vi "WPI_MotorControlScaleFromPWM.vi"(10 "Raw PWM Value":u8, 11 "DeadBand Info":T1={"Name"="", "maxPositivePwm"=0, "minPositivePwm"=0, "centerPwm"=0, "maxNegativePwm"=0, "minNegativePwm"=0, "angularRange"=170}) -> (2 "Output (1,-1)":dbl)   [LabVIEW 2017]
doc: "This software is licensed. Open the labview\\readme\\WPI Robotics Library Open Source License.txt file for more information."
uses:
  <vilib>/Rock Robotics/WPI/PWM/WPI_PWMDeadband.ctl
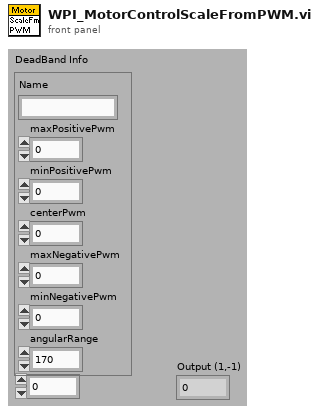
[diagram p1: front panel]
types:
  T1 = typedef "WPI_PWMDeadband.ctl" = cluster{"Name":string, "maxPositivePwm":i32, "minPositivePwm":i32, "centerPwm":i32, "maxNegativePwm":i32, "minNegativePwm":i32, "angularRange":u16}
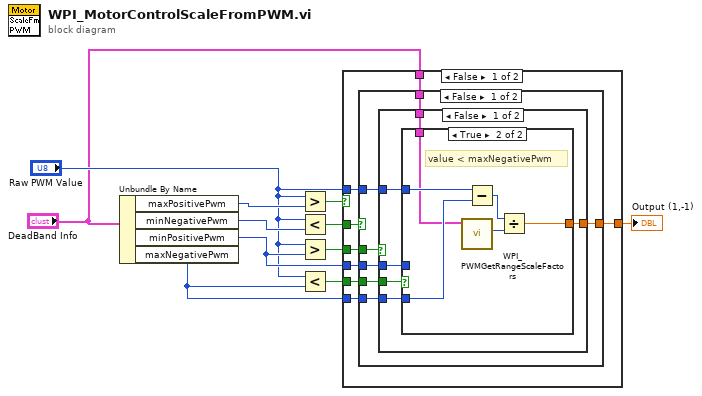
[diagram p0: block diagram]
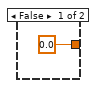
[diagram p2: hidden frame]
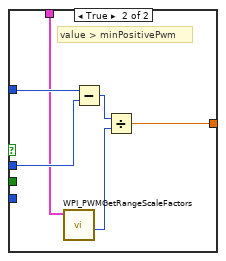
[diagram p3: hidden frame]
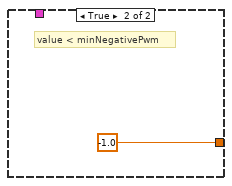
[diagram p4: hidden frame]
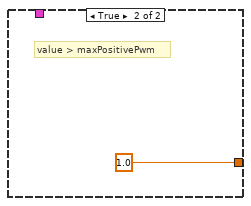
[diagram p5: hidden frame]
diagram:
  n1 = Unbundle By Name("DeadBand Info") -> ("maxPositivePwm"=w11:i32, "minNegativePwm"=w10:i32, "minPositivePwm"=w9:i32, "maxNegativePwm"=w8:i32)
  n2 = Greater?(x="Raw PWM Value", y=w11) -> (0:w4:bool)
  n3 = Less?(x="Raw PWM Value", y=w10) -> (x < y?=w5:bool)
  n4 = Greater?(x="Raw PWM Value", y=w9) -> (0:w6:bool)
  n5 = Less?(x="Raw PWM Value", y=w8) -> (x < y?=w7:bool)
  n6 = case shown="False" w4 {
    tunnel: "Raw PWM Value" -> [w19 _]
    tunnel: w9 -> [w18 _]
    tunnel: "DeadBand Info" -> [w17 _]
    tunnel: w8 -> [w16 _]
    tunnel: [w15 1.0] -> w1
    tunnel: w7 -> [w14 _]
    tunnel: w6 -> [w13 _]
    tunnel: w5 -> [w12 _]
    frame False {
      n7 = case shown="False" w12 {
        tunnel: w19 -> [w26 _]
        tunnel: w18 -> [w25 _]
        tunnel: w17 -> [w24 _]
        tunnel: w16 -> [w23 _]
        tunnel: [w22 -1.0] -> w15
        tunnel: w14 -> [w21 _]
        tunnel: w13 -> [w20 _]
        frame False {
          n8 = case shown="False" w20 {
            tunnel: w26 -> [w32 w44]
            tunnel: w25 -> [w31 w43]
            tunnel: w24 -> [w30 w41]
            tunnel: w23 -> [w29 _]
            tunnel: [w28 w42] -> w22
            tunnel: w21 -> [w27 _]
            frame False {
              n9 = case shown="True" w27 {
                tunnel: [0.0 w37] -> w28
                tunnel: w32 -> [_ w38]
                tunnel: w31 -> [_ _]
                tunnel: w30 -> [_ w35]
                tunnel: w29 -> [_ w36]
                frame False {
                }
                frame True {
                  # "value < maxNegativePwm"
                  n10 = call <vilib>:"WPI_PWMGetRangeScaleFactors.vi"("DeadBand"=w35) -> ("negativeScaleFactor"=w34:i32)  [unwired: 10 out]
                  n11 = Subtract(x=w38, y=w36) -> (x-y=w39:i32)
                  n12 = Divide(x=w39, y=w34) -> (x/y=w37:dbl)
                }
              }
            }
            frame True {
              # "value > minPositivePwm"
              n13 = call <vilib>:"WPI_PWMGetRangeScaleFactors.vi"("DeadBand"=w41) -> ("positiveScaleFactor"=w40:i32)  [unwired: 10 out]
              n14 = Subtract(x=w44, y=w43) -> (x-y=w45:i32)
              n15 = Divide(x=w45, y=w40) -> (x/y=w42:dbl)
            }
          }
        }
        frame True {
          # "value < minNegativePwm"
        }
      }
    }
    frame True {
      # "value > maxPositivePwm"
    }
  }
  "Output (1,-1)" <- w1
